vi "WSVCAP SHL Host TL I2C Write.vi"(0 "C1 Data Out":u8[][](array[numeric]) format="%.0x", 5 "C2 Data Out":u8[][](array[numeric]) format="%.0x", 7 "C3 Data Out":u8[][](array[numeric]) format="%.0x", 9 "Socket Mask Set [U64]":u64[](array[numeric]) format="%012x", 11 "error in":errorcluster, 12 "Sub Address":u8=20, 13 "Log (T)":bool=TRUE, 14 "FPGA":T1) -> (15 "error out":errorcluster)   [LabVIEW 2012]
uses:
  Type Defs/WSVCAP SHL I2C FPGA Enum.ctl
  Type Defs/WSVCAP SHL Function Enum.ctl
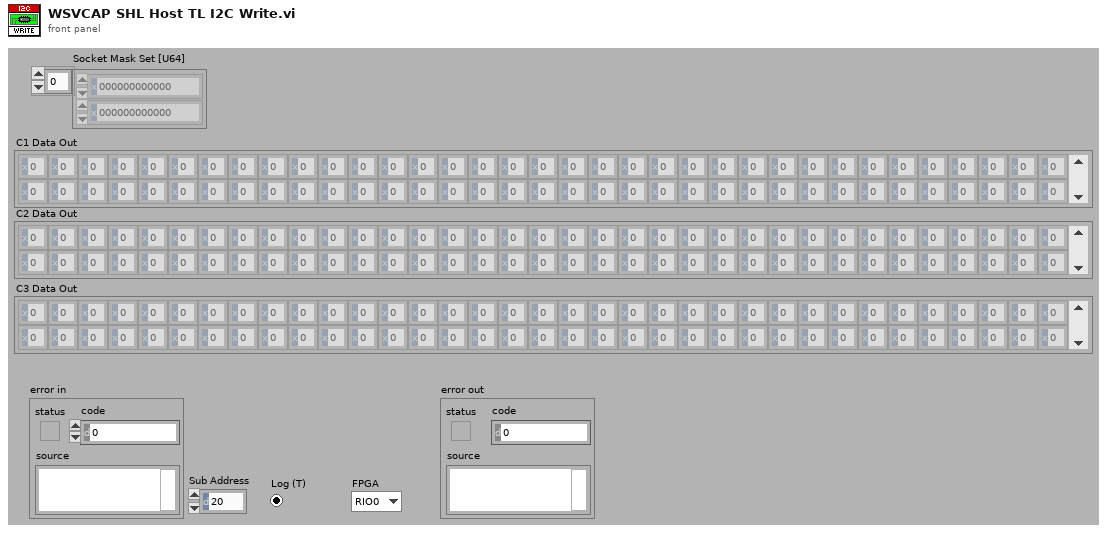
[diagram p1: front panel]
types:
  T1 = typedef "WSVCAP SHL I2C FPGA Enum.ctl" = enum16{"RIO0", "RIO1"}
  T2 = typedef "WSVCAP SHL Function Enum.ctl" = enum16{"Initialize", "Configure I2C", "Configure RFFE", "Write I2C", "Read I2C", "Write RFFE", "Read RFFE", "Start RFFE Cycle", "Stop RFFE Cycle", "Get Status", "Close"}
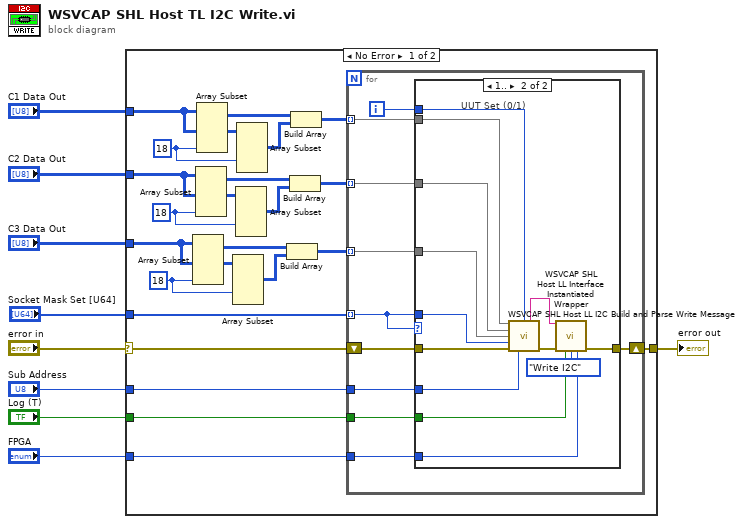
[diagram p0: block diagram]
diagram:
  n1 = case shown="No Error" "error in" {
    selector: "error in" -> [w29 w55]
    tunnel: [w30 w55] -> w9
    tunnel: "C1 Data Out" -> [w25 _]
    tunnel: "C2 Data Out" -> [w16 _]
    tunnel: "Sub Address" -> [w26 _]
    tunnel: "Socket Mask Set [U64]" -> [w28 _]
    tunnel: "Log (T)" -> [w27 _]
    tunnel: "C3 Data Out" -> [w13 _]
    tunnel: "FPGA" -> [w10 _]
    frame No Error {
      w18 = 18 ("length")
      w19 = 18 ("length")
      w24 = 18 ("length")
      n2 = Array Subset(array=w13, length (col)=w18) -> (w12:u8[][])  [unwired: 3 in]
      n3 = Array Subset(array=w16, length (col)=w19) -> (w15:u8[][])  [unwired: 3 in]
      n4 = Array Subset(array=w25, length (col)=w24) -> (w23:u8[][])  [unwired: 3 in]
      n5 = Array Subset(array=w13, index (col)=w18) -> (w17:u8[][])  [unwired: 3 in]
      n6 = Array Subset(array=w16, index (col)=w19) -> (w20:u8[][])  [unwired: 3 in]
      n7 = Array Subset(array=w25, index (col)=w24) -> (w22:u8[][])  [unwired: 3 in]
      n8 = Build Array(w12, w17) -> (w11:u8[][][])
      n9 = Build Array(w15, w20) -> (w14:u8[][][])
      n10 = Build Array(w23, w22) -> (w21:u8[][][])
      n11 = for {
        tunnel: w28 -> [w32] mode=indexing
        tunnel: w27 -> [w38]
        tunnel: w21 -> [w37] mode=indexing
        tunnel: w14 -> [w36] mode=indexing
        tunnel: w26 -> [w35]
        tunnel: w11 -> [w34] mode=indexing
        shift-right: [w40] -> w30
        shift-left: w29 -> [w39]
        tunnel: w10 -> [w31]
        i -> [w33]
        n12 = case shown="1.." w32 {
          tunnel: [w41 w53] -> w40
          tunnel: w39 -> [w41 w52]
          tunnel: w32 -> [_ w49]
          tunnel: w38 -> [_ w48]
          tunnel: w37 -> [_ w47]
          tunnel: w36 -> [_ w46]
          tunnel: w35 -> [_ w45]
          tunnel: w34 -> [_ w44]
          tunnel: w33 -> [_ w43]
          tunnel: w31 -> [_ w42]
          frame ..0 {
          }
          frame 1.. {
            # "UUT Set (0/1)"
            n13 = call "WSVCAP SHL Host LL I2C Build and Parse Write Message.vi"("C1 Write Data In [DUT Ordered]"=w47, "UUT Set (0/1) In"=w43, "C2 Write Data [DUT Ordered]"=w46, "C3Write Data [DUT Ordered]"=w44, "Socket Mask [U64] In"=w49, "error in"=w52, "Sub Address In"=w45) -> ("Message Out"=w50:string, "error out"=w51:errorcluster)  [unwired: 1 in, 6 out]
            n14 = call "WSVCAP SHL Host LL Interface Instantiated Wrapper.vi"("Message In"=w50, "error in"=w51, "Log (T)"=w48, "Function"=WSVCAP_SHL_Function_Enum."Write I2C", "FPGA"=w42) -> ("error out"=w53:errorcluster)  [unwired: 8 in, 2 out]
          }
        }
      }
    }
    frame Error {
    }
  }
  "error out" <- w9
